vi "Zdarzenie - filtracja.vi"() -> ()   [LabVIEW 2013]
doc: "Use this template to build a user interface event handler design pattern. Use this pattern for dialog boxes and other user interfaces. You also can create and execute user-defined events that the VI can handle the same way as user interface events."
panel:
  in  "Button 1":bool
  in  "stop":bool
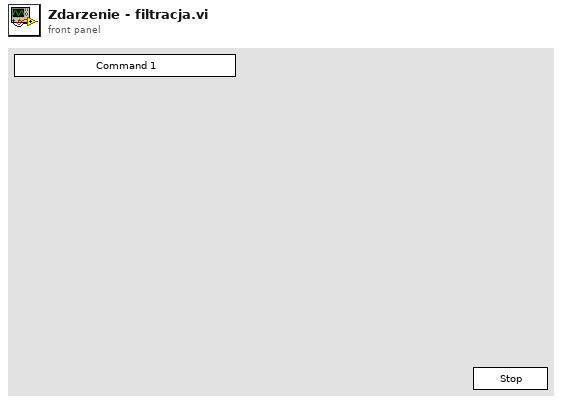
[diagram p1: front panel]
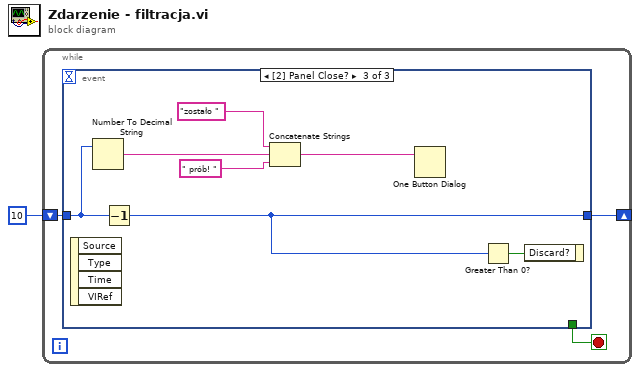
[diagram p0: block diagram]
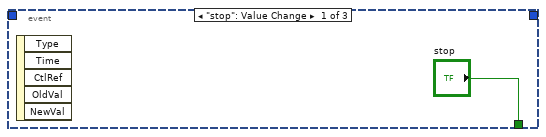
[diagram p2: hidden frame]
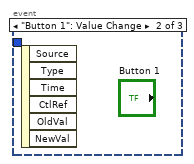
[diagram p3: hidden frame]
diagram:
  n1 = while {
    shift-right: [w2] -> _
    shift-left: 10 -> [w3]
    stop <- w4 stop-if-true
    n2 = event shown="[2] Panel Close?" {
      selector: _ -> [_ _ _]
      dyn-events: _ -> [_ _ _]
      timeout: _ -> [_ _ _]
      tunnel: ["stop" _ _] -> w4
      tunnel: w3 -> [_ _ w6]
      tunnel: [_ _ w7] -> w2
      event "stop": Value Change {
        n3 = event-data() -> ()  [unwired: 1 in, 5 out]
      }
      event "Button 1": Value Change {
        n4 = event-data() -> ()  [unwired: 1 in, 6 out]
      }
      event Panel Close? {
        n5 = event-data() -> ()  [unwired: 1 in, 4 out]
        n6 = Number To Decimal String(number=w6) -> (decimal integer string=w10:string)  [unwired: 1 in]
        n7 = Decrement(x=w6) -> (x-1=w7:i32)
        n8 = Concatenate Strings "Concatenate Strings"("zostało ", w10, " prób! ") -> (w8:string)
        n9 = One Button Dialog(message=w8) -> ()  [unwired: 1 in, 1 out]
        n10 = Greater Than 0?(x=w7) -> (x > 0?=w12:bool)
        n11 = event-data("Discard?"=w12) -> ()  [unwired: 1 in, 1 out]
      }
    }
  }
